vi "Clear_broken_frames_2_v16-Recalc_171213.vi"(11 "file path (dialog if empty)":path) -> (1 "Cleaned array":dbl[][](array[numeric]), 2 "Errors array":dbl[][](array[numeric]), 3 "Number of errors":i32)   [LabVIEW 2016]
uses:
  <vilib>/Utility/file.llb/Read Delimited Spreadsheet (DBL).vi
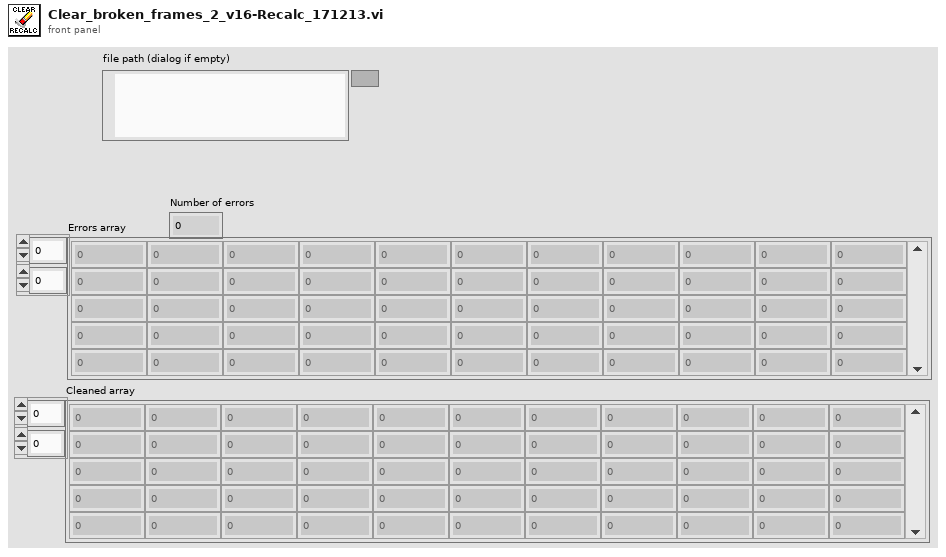
[diagram p1: front panel]
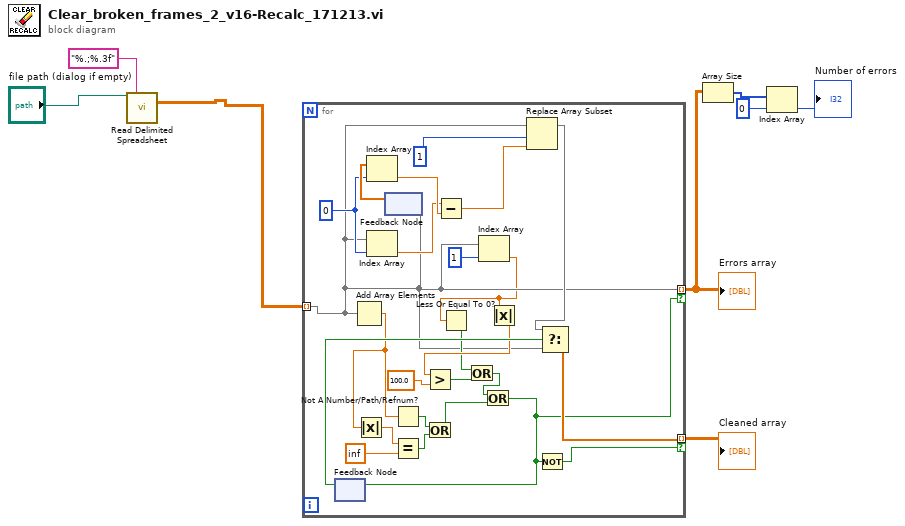
[diagram p0: block diagram]
diagram:
  n1 = call-poly <vilib>:"Read Delimited Spreadsheet.vi"("file path (dialog if empty)"="file path (dialog if empty)", "format (%.3f)"="%.;%.3f") -> ("all rows"=w2:dbl[][])  [unwired: 8 in, 5 out]
  n2 = for {
    tunnel: w2 -> [w11] mode=indexing
    tunnel: [w11] -> w5 mode=indexing if=w19
    tunnel: [w32] -> w4 mode=indexing if=w33
    w27 = 0 ("index")
    n3 = feedback #1() -> (w31:bool)  [unwired: 1 in]
    n4 = Add Array Elements(numeric array=w11) -> (sum=w21:dbl)
    n5 = Absolute Value(x=w21) -> (abs(x)=w20:dbl)
    n6 = Index Array(array=w11, index=w27) -> (element=w25:dbl)
    n7 = feedback #2() -> (w30:dbl[])  [unwired: 1 in]
    n8 = Index Array(array=w30, index=w27) -> (element=w26:dbl)
    n9 = feedback-in #2(w11) -> ()
    n10 = Not A Number/Path/Refnum?(number/path/refnum=w21) -> (NaN/Path/Refnum?=w24:bool)
    n11 = Equal?(x=w20, y=inf) -> (x = y?=w23:bool)
    n12 = Or(x=w24, y=w23) -> (x .or. y?=w18:bool)
    n13 = Subtract(x=w25, y=w26) -> (x-y=w13:dbl)
    n14 = Index Array(array=w11, index=1) -> (element=w9:dbl)
    n15 = Less Or Equal To 0?(x=w9) -> (x <= 0?=w12:bool)
    n16 = Absolute Value(x=w9) -> (abs(x)=w16:dbl)
    n17 = Greater?(x=w16, y=100.0) -> (0:w15:bool)
    n18 = Or(x=w12, y=w15) -> (x .or. y?=w14:bool)
    n19 = Or(x=w14, y=w18) -> (x .or. y?=w19:bool)
    n20 = feedback-in #1(w19) -> ()
    n21 = Replace Array Subset(array=w11, new element=w13, index=1) -> (w28:dbl[])
    n22 = Not(x=w19) -> (.not. x?=w33:bool)
    n23 = Select(t=w28, s=w31, f=w11) -> (s? t:f=w32:dbl[])
  }
  "Errors array" <- w5
  "Cleaned array" <- w4
  n24 = Array Size(array=w5) -> (size(s)=w6:i32[])
  n25 = Index Array(array=w6, index=0) -> (element=→"Number of errors":i32)
